vi "FABR-Update Display.vi"(0 "Analysis in":T1, 7 "finished":bool, 9 "Normalize traces":bool, 11 "error in (no error)":errorcluster, 12 "scale":dbl, 13 "Cluster":T3) -> (4 "Analysis thru":T1, 15 "error out":errorcluster)   [LabVIEW 2020]
uses:
  Typedefs/FABR-Analysis State.ctl
  Threshold Estimation VIs/ABR3-Threshold Estimation Result.ctl
panel:
  # "Freq X Level X Time"
  # "Freq X Level X Time"
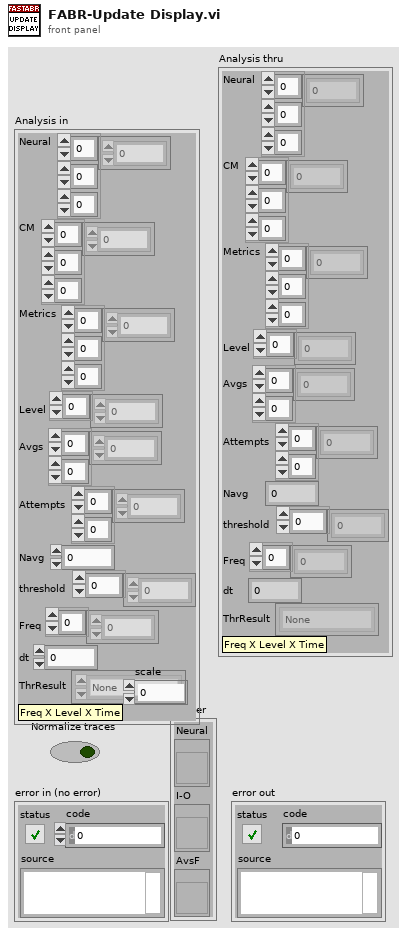
[diagram p1: front panel]
types:
  T1 = typedef "FABR-Analysis State.ctl" = cluster{"Neural":dbl[][][], "CM":dbl[][][], "Metrics":dbl[][][], "Level":dbl[], "Avgs":i32[][], "Attempts":i32[][], "Navg":i32, "threshold":dbl[], "Freq":dbl[], "dt":dbl, "ThrResult":T2[]}
  T2 = typedef "ABR3-Threshold Estimation Result.ctl" = enum16{"None", "Power", "Sigmoid", "Power (noisy)", "Suprathreshold", "Invalid"}
  T3 = cluster{"Neural":refnum<vi>, "I-O":refnum<vi>, "AvsF":refnum<vi>}
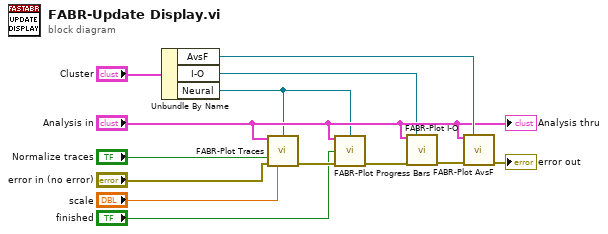
[diagram p0: block diagram]
diagram:
  n1 = Unbundle By Name("Cluster") -> ("AvsF"=w9:refnum<vi>, "I-O"=w4:refnum<vi>, "Neural"=w3:refnum<vi>)
  n2 = call "FABR-Plot Traces.vi"("Analysis"="Analysis in", "Neural Ref"=w3, "Normalize individual?"="Normalize traces", "error in (no error)"="error in (no error)", "Scale"="scale") -> ("error out"=w7:errorcluster)  [unwired: 10 in]
  n3 = call "FABR-Plot Progress Bars.vi"("Analysis"="Analysis in", "Neural Ref"=w3, "finished"="finished", "error in (no error)"=w7) -> ("error out"=w6:errorcluster)  [unwired: 11 in]
  n4 = call "FABR-Plot I-O.vi"("Analysis"="Analysis in", "I-O"=w4, "error in (no error)"=w6) -> ("error out"=w10:errorcluster)  [unwired: 12 in]
  n5 = call "FABR-Plot AvsF.vi"("Analysis"="Analysis in", "I-O"=w9, "error in (no error)"=w10) -> ("error out"=→"error out":errorcluster)  [unwired: 12 in]
  "Analysis thru" <- "Analysis in"
